vi "Get VI Icon and Save to PNG(冲突时的文件备份2013-03-27 14-09-02).vi"(8 "错误输入（无错误）":errorcluster, 11 "VI Path":path) -> (0 "错误输出":errorcluster)   [LabVIEW 2012, in "Application.lvlib"]
uses:
  Application.lvlib
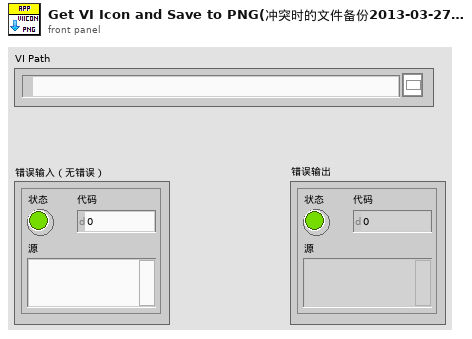
[diagram p1: front panel]
types:
  T1 = typedef "imagedata.ctl" = cluster{"image type":i32, "image depth":i32, "image":u8[], "mask":u8[], "colors":u32[], "Rectangle":cluster{"left":i16, "top":i16, "right":i16, "bottom":i16}}
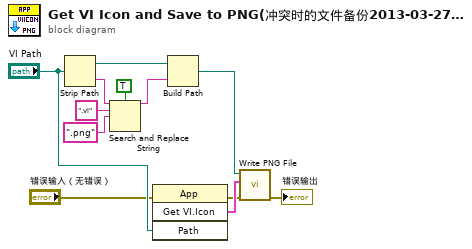
[diagram p0: block diagram]
diagram:
  n1 = Strip Path(path="VI Path") -> (stripped path=w7:path, name=w10:string)
  n2 = Search and Replace String(case sensitive?=TRUE ("忽略大小写？(F)"), input string=w10, search string=".vi" ("搜索字符串"), replace string=".png" ("替换字符串(\"\")")) -> (result string=w6:string)  [unwired: 4 in, 3 out]
  n3 = invoke class="App" method="Get VI.Icon"(error in="错误输入（无错误）", "Path"="VI Path") -> (error out=w2:errorcluster, "Get VI.Icon"=w12:T1)  [unwired: 2 in, 2 out]
  n4 = Build Path(base path=w7, name or relative path=w6) -> (appended path=w4:path)
  n5 = call <vilib>:"Write PNG File.vi"("error in (no error)"=w2, "image data"=w12, "path to PNG file"=w4) -> ("error out"=→"错误输出":errorcluster)  [unwired: 7 in, 1 out]
